vi "StopConnection.vi"(8 "ErrorIn":errorcluster, 11 "Reference":T1) -> (0 "ErrorOut":errorcluster)   [LabVIEW 2019]
uses:
  C:/Users/yasav/Downloads/prev_robocad/robocadSimLVFolder/assemblies/LibraryForLabVIEW.dll
  assemblies/LibraryForLabVIEW.dll
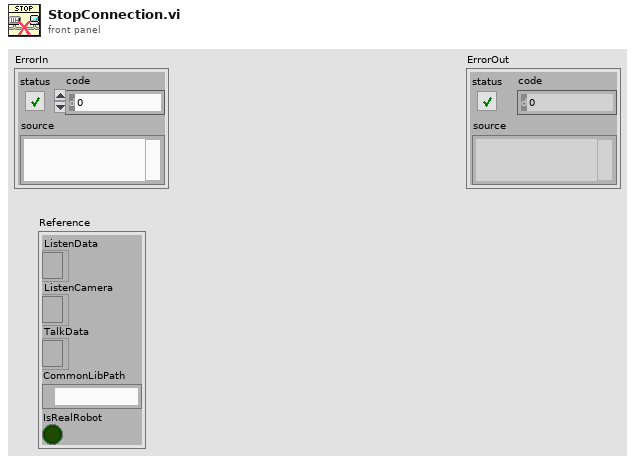
[diagram p1: front panel]
types:
  T1 = cluster{"ListenData":refnum<k24>, "ListenCamera":refnum<k24>, "TalkData":refnum<k24>, "CommonLibPath":path, "IsRealRobot":bool}
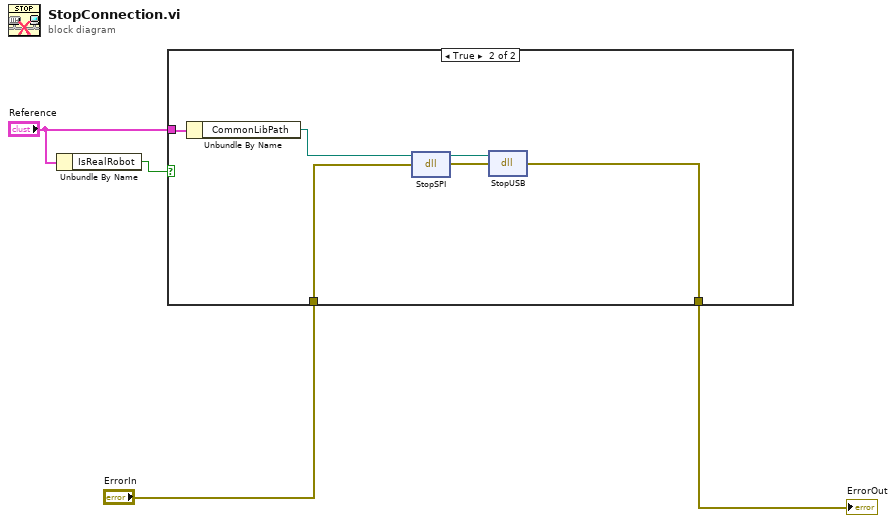
[diagram p0: block diagram]
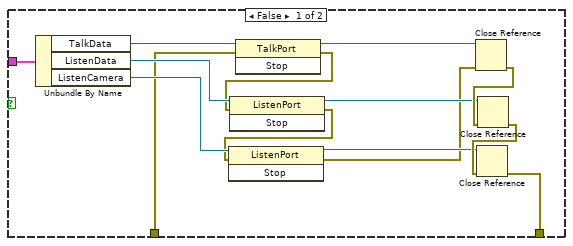
[diagram p2: hidden frame]
diagram:
  n1 = Unbundle By Name("Reference") -> ("IsRealRobot"=w1:bool)
  n2 = case shown="True" w1 {
    tunnel: "ErrorIn" -> [w10 w20]
    tunnel: [w6 w19] -> w3
    tunnel: "Reference" -> [w5 w22]
    frame False {
      n3 = Unbundle By Name(w5) -> ("TalkData"=w11:refnum<k24>, "ListenData"=w18:refnum<k24>, "ListenCamera"=w17:refnum<k24>)
      n4 = invoke class="TalkPort" method="Stop"(reference=w11, error in=w10) -> (reference out=w9:refnum<k24>, error out=w8:errorcluster)  [unwired: 1 in, 1 out]
      n5 = invoke class="ListenPort" method="Stop"(reference=w18, error in=w8) -> (reference out=w14:refnum<k24>, error out=w16:errorcluster)  [unwired: 1 in, 1 out]
      n6 = invoke class="ListenPort" method="Stop"(reference=w17, error in=w16) -> (reference out=w12:refnum<k24>, error out=w7:errorcluster)  [unwired: 1 in, 1 out]
      n7 = Close Reference(reference=w9, error in (no error)=w7) -> (error out=w15:errorcluster)
      n8 = Close Reference(reference=w14, error in (no error)=w15) -> (error out=w13:errorcluster)
      n9 = Close Reference(reference=w12, error in (no error)=w13) -> (error out=w6:errorcluster)
    }
    frame True {
      n10 = Unbundle By Name(w22) -> ("CommonLibPath"=w21:path)
      n11 = dll-call lib="?" fn="StopSPI"(path in=w21, error in=w20) -> (path out=w24:path, error out=w23:errorcluster)  [unwired: 2 in]
      n12 = dll-call lib="?" fn="StopUSB"(path in=w24, error in=w23) -> (error out=w19:errorcluster)  [unwired: 2 in, 1 out]
    }
  }
  "ErrorOut" <- w3
